vi "Get Errors.vi"(8 "error in (no error)":errorcluster, 11 "Command Execution in":refnum<class "Command Execution.lvclass">) -> (0 "error out":errorcluster, 2 "Errors":T1[](array[typedef]), 3 "Command Execution out":refnum<class "Command Execution.lvclass">)   [LabVIEW 2015, in "WinSCP.lvlib" / "Command Execution.lvclass"]
uses:
  Command Execution.lvclass
  ErrorDescription.ctl
  Command Execution.lvclass/Command Execution.ctl
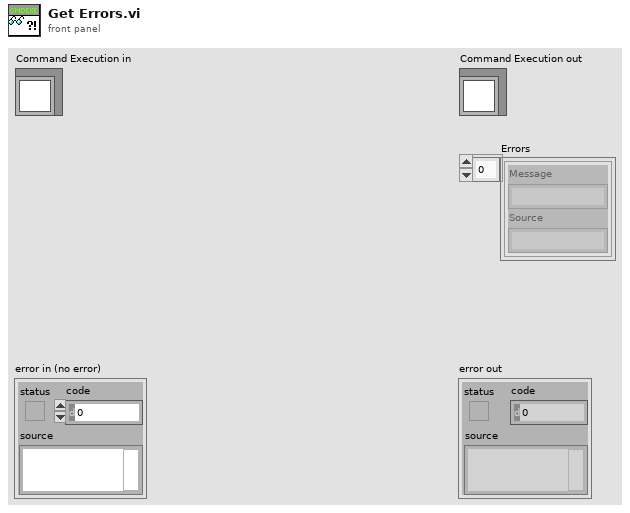
[diagram p1: front panel]
types:
  T1 = typedef "WinSCP.lvlib/Command Execution.lvclass/ErrorDescription.ctl" = cluster{"Message":string, "Source":string}
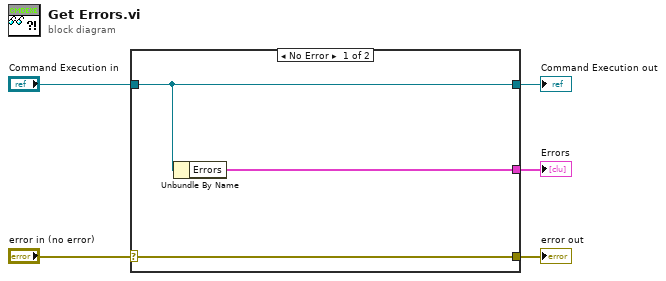
[diagram p0: block diagram]
diagram:
  n1 = case shown="No Error" "error in (no error)" {
    selector: "error in (no error)" -> [w8 w9]
    tunnel: [w8 w9] -> w4
    tunnel: [w7 w10] -> w2
    tunnel: "Command Execution in" -> [w7 w10]
    tunnel: [w6 _] -> w1
    frame No Error {
      n2 = Unbundle By Name(w7) -> ("Errors"=w6:T1[])
    }
    frame Error {
    }
  }
  "error out" <- w4
  "Command Execution out" <- w2
  "Errors" <- w1
